vi "get Alarms.vi"(10 "alrm":u64, 11 "devID":u32) -> (2 "alrm out":u64, 3 "function return":i32)   [LabVIEW 2014, in "libchaos-driver-powersupply-labview.lvlib"]
doc: "int getAlarms(unsigned int devID,long long *alrm);"
uses:
  libchaos-driver-powersupply-labview.lvlib
  chaos-i686-dynamic-release/lib/libchaos-driver-powersupply-labview.so
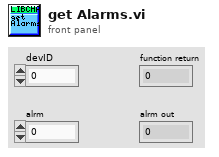
[diagram p1: front panel]
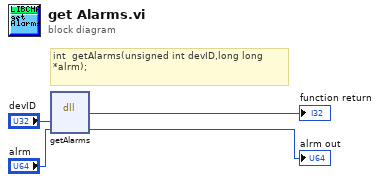
[diagram p0: block diagram]
diagram:
  # "int  getAlarms(unsigned int devID,long long *alrm);"
  n1 = dll-call lib="home/chaos/chaos_bundle/chaos-i686-dynamic-release/lib/libchaos-driver-powersupply-labview.*" fn="getAlarms"("devID"="devID", "alrm"="alrm") -> (→"function return":i32, "alrm"=→"alrm out":u64)  [unwired: 4 in, 2 out]
